vi "subvi_ArrayToBytes.vi"(5 "Endian-ness (T, Big)":bool=TRUE, 7 "#pragma directive (0, default)":i32, 8 "error in (no error)":errorcluster, 9 "data string":string, 10 "Dims \"N\"":i16, 11 "type string":i16[](array[numeric])) -> (0 "error out":errorcluster, 1 "Element Sizes":i32[](array[numeric]), 2 "Data Element Algnment Target":i32[](array[numeric]), 3 "Cluster Data as Byte Array Out":u8[](array[numeric]), 4 "Data Mask":bool[](array[boolean]), 6 "Base Data Element Info":T1[](array[typedef]))   [LabVIEW 2020]
uses:
  TypeDefs/ctl_DataElementInfo.ctl
panel:
  # "### BSD License (http://www.opensource.org/licenses/bsd-license.php) Begin ###\n \nCopyright (c) 2014 Jeffrey Holt <jolt.holt@gmail.com>\n\nAll rights reserved.\n\nRedistribution and use in source and binary forms, with or without modification, are permitted provided that the following conditions are met:\n\n    * Redistributions of source code must retain the above copyright notice\n\nTHIS SOFTWARE IS PROVIDED BY THE COPYRIGHT HOLDERS AND CONTRIBUTORS \"AS IS\" AND ANY EXPRESS OR IMPLIED WARRANTIES, \nINCLUDING, BUT NOT LIMITED TO, THE IMPLIED WARRANTIES OF MERCHANTABILITY AND FITNESS FOR A PARTICULAR PURPOSE ARE \nDISCLAIMED. IN NO EVENT SHALL THE COPYRIGHT OWNER OR CONTRIBUTORS BE LIABLE FOR ANY DIRECT, INDIRECT, INCIDENTAL,\n SPECIAL, EXEMPLARY, OR CONSEQUENTIAL DAMAGES (INCLUDING, BUT NOT LIMITED TO, PROCUREMENT OF SUBSTITUTE GOODS OR \nSERVICES; LOSS OF USE, DATA, OR PROFITS; OR BUSINESS INTERRUPTION) HOWEVER CAUSED AND ON ANY THEORY OF LIABILITY, \nWHETHER IN CONTRACT, STRICT LIABILITY, OR TORT (INCLUDING NEGLIGENCE OR OTHERWISE) ARISING IN ANY WAY OUT OF THE USE \nOF THIS SOFTWARE, EVEN IF ADVISED OF THE POSSIBILITY OF SUCH DAMAGE.\n\n### BSD License End ###"
  # "Parts of this code was adapted from:\n\nGet Array Element TD.vi\n\nPlease visit http://www.OpenG.org to learn about the\nOpen Source LabVIEW software movement.\n\nNOTICE -- YOU MUST LEAVE THIS NOTICE IN PLACE.  PER THE TERMS OF THE LICENSE BELOW, YOU MAY SUBLICENSE THIS SOFTWARE \nIN ANY WAY THAT DOES NOT CONFLICT WITH THIS LICENSE.\n\n### BSD License (http://www.opensource.org/licenses/bsd-license.php) Begin ###\n \nCopyright (c) 2002, Jean-Pierre Drolet <drolet_jp@hotmail.com>\nCopyright (c) 2002-2006, Jim Kring <jim@jimkring.com>\n\nAll rights reserved.\n\nRedistribution and use in source and binary forms, with or without modification, are permitted provided that the following conditions are met:\n\n    * Redistributions of source code must retain the above copyright notice, this list of conditions and the following disclaimer.\n    * Redistributions in binary form must reproduce the above copyright notice, this list of conditions and the following disclaimer in the \n       documentation and/or other materials provided with the distribution.\n    * Neither the name of SciWare, James Kring, Inc., nor the names of its contributors may be used to endorse or promote products derived \n       from this software without specific prior written permission.\n\nTHIS SOFTWARE IS PROVIDED BY THE COPYRIGHT HOLDERS AND CONTRIBUTORS \"AS IS\" AND ANY EXPRESS OR IMPLIED WARRANTIES, \nINCLUDING, BUT NOT LIMITED TO, THE IMPLIED WARRANTIES OF MERCHANTABILITY AND FITNESS FOR A PARTICULAR PURPOSE ARE \nDISCLAIMED. IN NO EVENT SHALL THE COPYRIGHT OWNER OR CONTRIBUTORS BE LIABLE FOR ANY DIRECT, INDIRECT, INCIDENTAL,\n SPECIAL, EXEMPLARY, OR CONSEQUENTIAL DAMAGES (INCLUDING, BUT NOT LIMITED TO, PROCUREMENT OF SUBSTITUTE GOODS OR \nSERVICES; LOSS OF USE, DATA, OR PROFITS; OR BUSINESS INTERRUPTION) HOWEVER CAUSED AND ON ANY THEORY OF LIABILITY, \nWHETHER IN CONTRACT, STRICT LIABILITY, OR TORT (INCLUDING NEGLIGENCE OR OTHERWISE) ARISING IN ANY WAY OUT OF THE USE \nOF THIS SOFTWARE, EVEN IF ADVISED OF THE POSSIBILITY OF SUCH DAMAGE.\n\n### BSD License End ###"
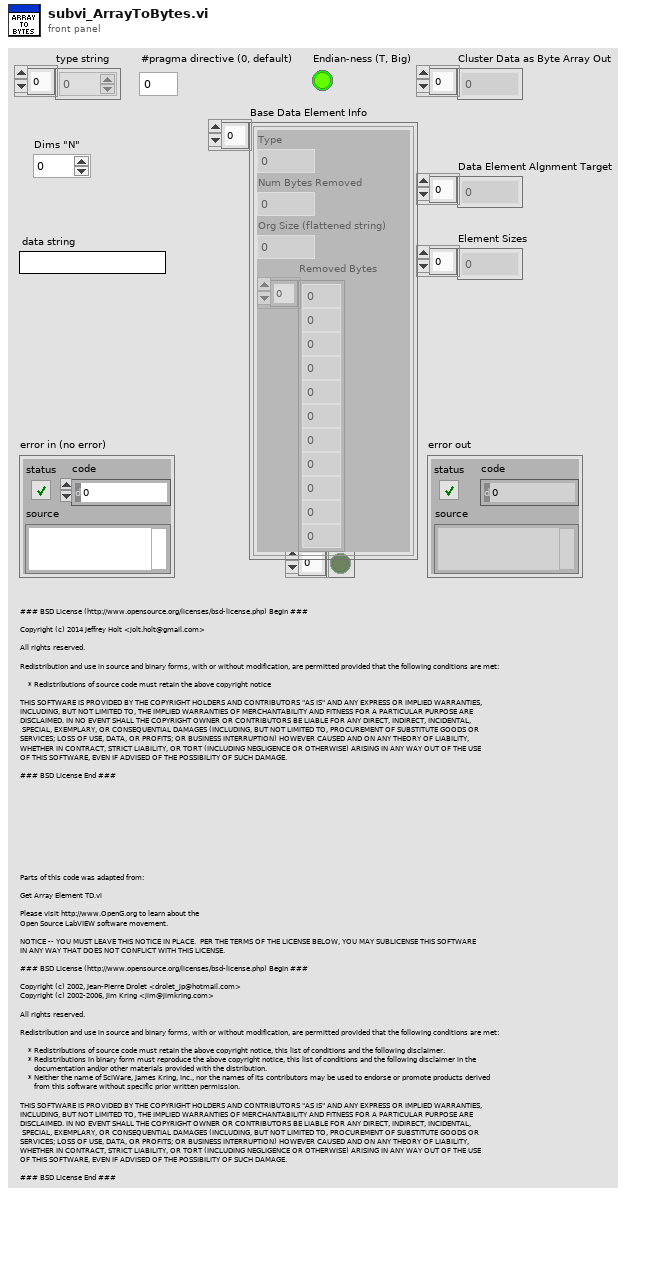
[diagram p1: front panel]
types:
  T1 = typedef "ctl_DataElementInfo.ctl" = cluster{"Type":u16, "Num Bytes Removed":u16, "Org Size (flattened string)":i32, "Removed Bytes":u8[]}
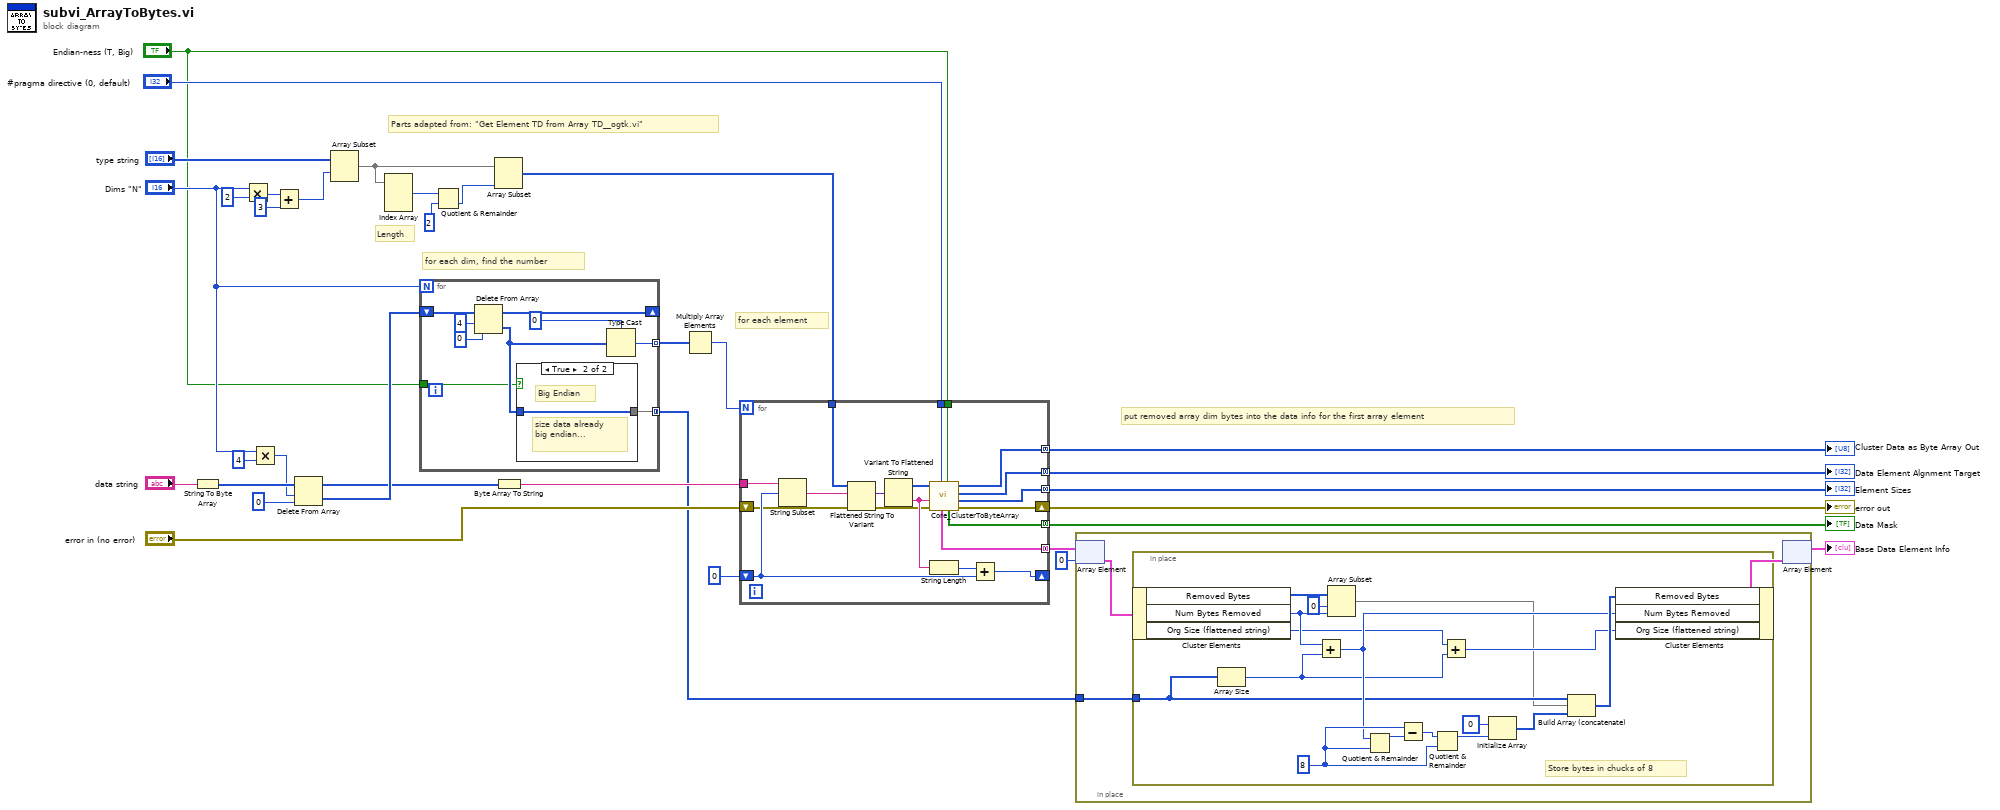
[diagram p0: block diagram]
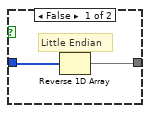
[diagram p2: hidden frame]
diagram:
  # "put removed array dim bytes into the data info for the first array element"
  # "for each element"
  # "for each dim, find the number"
  # "Parts adapted from: \"Get Element TD from Array TD__ogtk.vi\""
  # "Length"
  n1 = String To Byte Array(string="data string") -> (unsigned byte array=w23:u8[])
  n2 = Multiply(x="Dims \"N\"", y=2) -> (x*y=w17:i32)
  n3 = Multiply(x="Dims \"N\"", y=i16 4) -> (x*y=w22:i16)
  n4 = Add(x=w17, y=3) -> (x+y=w19:i32)
  n5 = Delete From Array(array=w23, length=w22, index=0) -> (deleted portion=w27:u8[], array with subset deleted=w24:u8[])
  n6 = Array Subset(array="type string", index=w19) -> (w14:i16[])  [unwired: 1 in]
  n7 = Index Array(array=w14) -> (element #1=w15:i16)  [unwired: 3 in, 2 out]
  n8 = for {
    N: "Dims \"N\"" -> [_]
    shift-right: [w42] -> _
    shift-left: w27 -> [w43]
    tunnel: [w38] -> w26 mode=indexing
    tunnel: "Endian-ness (T, Big)" -> [w36]
    tunnel: [w35] -> w1 mode=concatenating
    n9 = Delete From Array(array=w43, length=4, index=0) -> (deleted portion=w37:u8[], array with subset deleted=w42:u8[])
    n10 = case shown="True" w36 {
      tunnel: [w44 w46] -> w35
      tunnel: w37 -> [w45 w46]
      frame False {
        # "Little Endian"
        n11 = Reverse 1D Array(array=w45) -> (reversed array=w44:u8[])
      }
      frame True {
        # "Big Endian"
        # "size data already big endian..."
      }
    }
    n12 = Type Cast(type=0, x=w37) -> (*(type *) &x=w38:i32)
  }
  n13 = Quotient & Remainder(x=w15, y=u16 2) -> (floor(x/y)=w12:u16)  [unwired: 1 out]
  n14 = Array Subset(array=w14, length=w12) -> (w29:i16[])  [unwired: 1 in]
  n15 = Byte Array To String(unsigned byte array=w24) -> (string=w31:string)
  n16 = Multiply Array Elements(1:w26) -> (0:w28:i32)
  n17 = for {
    N: w28 -> [_]
    tunnel: w29 -> [w63]
    tunnel: w31 -> [w64]
    shift-right: [w60] -> _
    shift-left: 0 ("Offset In") -> [w61]
    tunnel: [w56] -> w33 mode=concatenating
    tunnel: [w55] -> w34 mode=concatenating
    tunnel: "Endian-ness (T, Big)" -> [w54]
    tunnel: "#pragma directive (0, default)" -> [w53]
    tunnel: [w52] -> w8 mode=concatenating
    tunnel: [w51] -> w9 mode=concatenating
    shift-right: [w48] -> w6
    shift-left: "error in (no error)" -> [w49]
    tunnel: [w47] -> w4 mode=concatenating
    n18 = String Subset(string=w64, offset (0)=w61) -> (substring=w59:string)  [unwired: 1 in]
    n19 = Flattened String To Variant(4:w49, 6:w59, 7:w63) -> (0:w50:errorcluster, 3:w65:variant)
    n20 = Variant To Flattened String(Variant=w65) -> (data string=w57:string, 1:w58:i16[])
    n21 = call "Core_ClusterToByteArray.vi"("Endian-ness (T, Big)"=w54, "#pragma directive (0, default)"=w53, "error in (no error)"=w50, "data string (big endian)"=w57, "type string"=w58) -> ("error out"=w48:errorcluster, "Element Sizes (used in padding calculation)"=w51:i32[], "Data Element Algnment Target"=w52:i32[], "Cluster Data as Byte Array Out"=w56:u8[], "Data Mask"=w55:bool[], "Base Data Element Info"=w47:T1[])  [unwired: 1 in]
    n22 = String Length(string=w57) -> (length=w62:i32)
    n23 = Add(x=w62, y=w61) -> (x+y=w60:i32)
  }
  "Data Mask" <- w34
  "Cluster Data as Byte Array Out" <- w33
  "Element Sizes" <- w9
  "Data Element Algnment Target" <- w8
  "error out" <- w6
  n24 = in-place {
    in-place-border: w1 -> [w67]
    n25 = in-place-array #1(w4, 0) -> (w68:T1)
    n26 = in-place {
      in-place-border: w67 -> [w70]
      w79 = 8 ("y")
      # "Store bytes in chucks of 8"
      n27 = in-place-cluster #2(w68) -> ("Removed Bytes"=w84:u8[], "Num Bytes Removed"=w82:u16, "Org Size (flattened string)"=w73:i32)
      n28 = Array Size(array=w70) -> (size(s)=w72:i32)
      n29 = Add(x=w82, y=w72) -> (x+y=w74:i32)
      n30 = Array Subset(array=w84, index=0, length=w82) -> (w69:u8[])
      n31 = Quotient & Remainder(x=w74, y=w79) -> (x-y*floor(x/y)=w81:i32)  [unwired: 1 out]
      n32 = Subtract(x=w79, y=w81) -> (x-y=w80:i32)
      n33 = Quotient & Remainder(x=w80, y=w79) -> (x-y*floor(x/y)=w77:i32)  [unwired: 1 out]
      n34 = Add(x=w73, y=w72) -> (x+y=w71:i32)
      n35 = Initialize Array(u8 0, w77) -> (w76:u8[])
      n36 = Build Array (concatenate)(w70, w69, w76) -> (w75:u8[])
      n37 = in-place-cluster #2("Removed Bytes"=w75, "Num Bytes Removed"=w74, "Org Size (flattened string)"=w71) -> (w66:T1)
    }
    n38 = in-place-array #1(w66) -> (→"Base Data Element Info":T1[])  [unwired: 1 out]
  }
